vi "DAQmx test.vi"() -> ()   [LabVIEW 2017]
uses:
  <vilib>/DAQmx/write.llb/DAQmx Write (Analog 2D DBL NChan NSamp).vi
  <vilib>/DAQmx/create/channels.llb/DAQmx Create Channel (AO-Voltage-Basic).vi
  <vilib>/DAQmx/configure/timing.llb/DAQmx Timing (Sample Clock).vi
  <vilib>/DAQmx/miscellaneous.llb/DAQmx Fill In Error Info.vi
panel:
  out "error out":errorcluster
  in  "error in":errorcluster
  in  "Voltage data":dbl[][](array[numeric]) format="%0.2f"
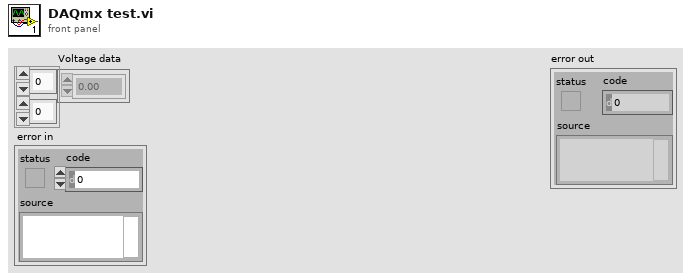
[diagram p1: front panel]
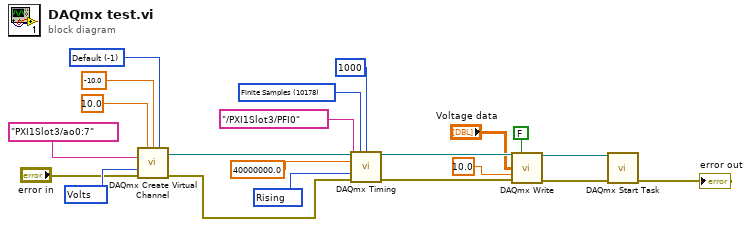
[diagram p0: block diagram]
diagram:
  w11 = 10178 items=["Finite Samples"=10178, "Continuous Samples"=10123, "Hardware Timed Single Point"=12522] ("sample mode")
  w13 = 10280 items=["Rising"=10280, "Falling"=10171] ("active edge")
  w18 = 10348 items=["Volts"=10348, "From Custom Scale"=10065] ("units")
  w19 = -1 items=["Default"=-1, "RSE"=10083, "Differential"=10106, "Pseudodifferential"=12529] ("output terminal configuration")
  n1 = call-poly <vilib>:"DAQmx Create Virtual Channel.vi"("maximum value"=10.0, "minimum value"=-10.0, "output terminal configuration"=w19, "physical channels"=tag "PXI1Slot3/ao0:7", "units"=w18, "error in"="error in") -> ("task out"=w16:refnum<k21>, "error out"=w7:errorcluster)  [unwired: 8 in]
  n2 = call-poly <vilib>:"DAQmx Timing.vi"("task/channels in"=w16, "sample mode"=w11, "samples per channel"=1000, "rate"=40000000.0, "source"=tag "/PXI1Slot3/PFI0", "active edge"=w13, "error in"=w7) -> ("task out"=w10:refnum<k21>, "error out"=w6:errorcluster)  [unwired: 7 in]
  n3 = call-poly <vilib>:"DAQmx Write.vi"("task/channels in"=w10, "auto start"=FALSE, "data"="Voltage data", "timeout"=10.0, "error in"=w6) -> ("task out"=w3:refnum<k21>, "error out"=w2:errorcluster)  [unwired: 8 in, 1 out]
  n4 = call <vilib>:"DAQmx Start Task.vi"("task/channels in"=w3, "error in"=w2) -> ("error out"=→"error out":errorcluster)  [unwired: 12 in, 1 out]
